vi "nominal video property key at.vi"(6 "out_needed":u32, 7 "cap":u32, 8 "error in (no error)":errorcluster, 9 "buf":string, 10 "index":i32, 11 "video":i32) -> (0 "error out":errorcluster, 1 "buf out":string, 3 "function return":i32, 4 "out_needed out":u32)   [LabVIEW 2020, in "client.lvlib"]
doc: "int32_t nominal_video_property_key_at(int32_t video,\n int32_t index,\n char *buf,\n uint32_t cap,\n uint32_t *out_needed);"
uses:
  client.lvlib
  nominalClient_64.dll
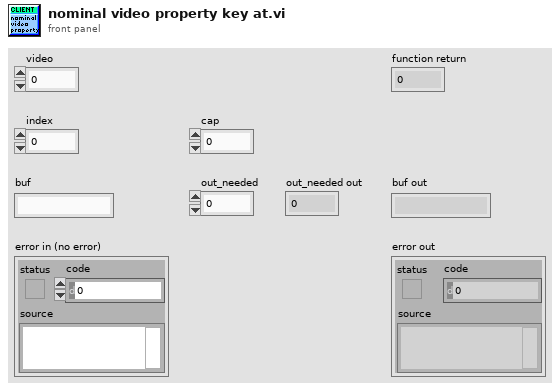
[diagram p1: front panel]
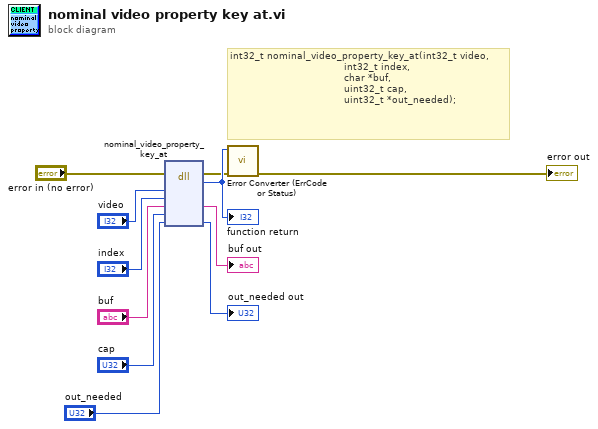
[diagram p0: block diagram]
diagram:
  # "int32_t nominal_video_property_key_at(int32_t video,\n                                      int32_t index,\n                                      char *buf,\n                                      uint32_t cap,\n                                      uint32_t *out_needed);"
  n1 = dll-call lib="C:/code/labview-client-rs/lv_src/client/nominalClient_*.*" fn="nominal_video_property_key_at"(error in="error in (no error)", "video"="video", "index"="index", "buf"="buf", "cap"="cap", "out_needed"="out_needed") -> (error out=w2:errorcluster, w11:i32, "buf"=→"buf out":string, "out_needed"=→"out_needed out":u32)  [unwired: 5 in, 1 out]
  "function return" <- w11
  n2 = call "Error Converter (ErrCode or Status).vi"("error in (no error)"=w2, "error code"=w11) -> ("error out"=→"error out":errorcluster)  [unwired: 9 in]
